vi "XY Graph Set Plot Style.vi"(8 "Error In":errorcluster, 9 "Plot Index (0)":i32, 10 "Single Plot Style":T1, 11 "XY Graph Refnum in":refnum<vi>) -> (0 "Error Out":errorcluster, 3 "XY Graph Refnum out":refnum<vi>)   [LabVIEW 2019, in "XY Graph Add-Ons.lvlib"]
uses:
  XY Graph Add-Ons.lvlib
  Single Plot Style 2.ctl
  Plot Style Settings Step.ctl
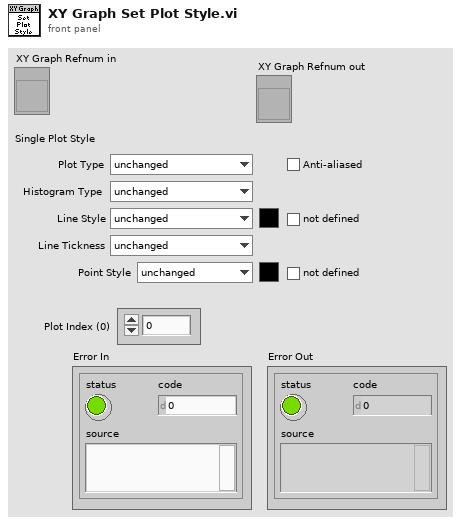
[diagram p1: front panel]
types:
  T1 = typedef "Single Plot Style 2.ctl" = cluster{"Plot Style":enum16{"unchanged", "Line", "Symbol", "Line + Symbol", "Histogram", "Histogram + Symbol"}, "Histogram Type":enum16{"unchanged", "Left Bound", "Center", "Right Bound"}, "Line Tickness":enum16{"unchanged", "Thin", "1 pixel", "2 pixel", "3 pixel", "4 pixel", "5 pixel"}, "Line Style":enum16{"unchanged", "Plain", "Long Dash", "Short Dash", "Long-Short Dash", "Long-Short-Short Dash"}, "Point Style":enum16{"unchanged", "None", "Empty Circle", "Filled Circle", "Thick Circle", "Dotted Circle", "Empty Square", "Filled Square", "Thick Square", "Dotted Square", "Small Filled Square", "Dot", "Cross", "Tiny Cross", "Large X", "Small x", "Diamond", "Small Empty Square"}, "Line Color":u32, "Line Color defined?":bool, "Point Color":u32, "Point Color defined?":bool, "Anti-aliased":bool}
  T2 = typedef "Plot Style Settings Step.ctl" = enum16{"Plot Type", "Line Style", "Line Thickness", "Line Color", "Point Style", "Point Color", "Aliasing"}
  T3 = enum16{"unchanged", "Line", "Symbol", "Line + Symbol", "Histogram", "Histogram + Symbol"}
  T4 = enum16{"unchanged", "Left Bound", "Center", "Right Bound"}
  T5 = enum16{"unchanged", "Plain", "Long Dash", "Short Dash", "Long-Short Dash", "Long-Short-Short Dash"}
  T6 = enum16{"unchanged", "Thin", "1 pixel", "2 pixel", "3 pixel", "4 pixel", "5 pixel"}
  T7 = enum16{"unchanged", "None", "Empty Circle", "Filled Circle", "Thick Circle", "Dotted Circle", "Empty Square", "Filled Square", "Thick Square", "Dotted Square", "Small Filled Square", "Dot", "Cross", "Tiny Cross", "Large X", "Small x", "Diamond", "Small Empty Square"}
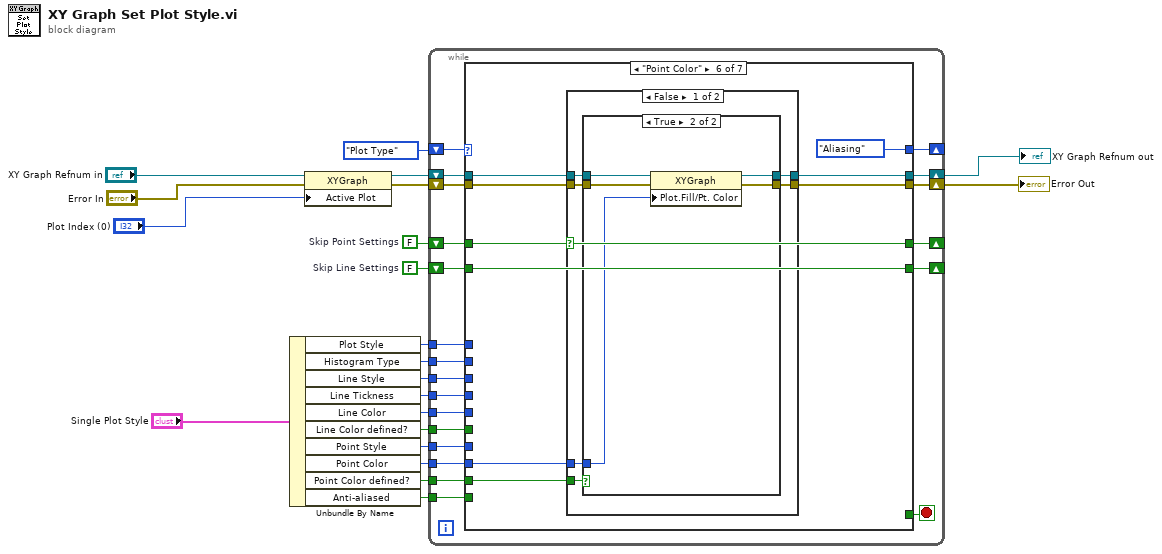
[diagram p0: block diagram]
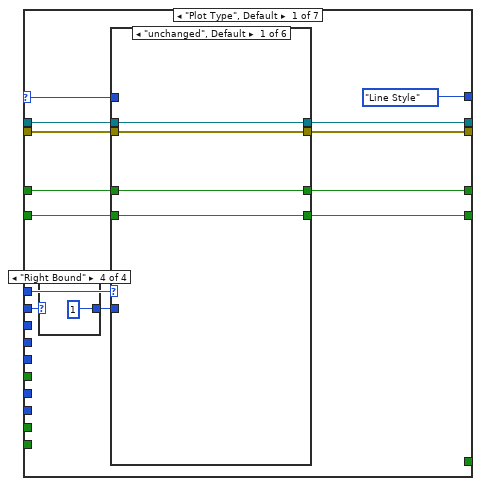
[diagram p2: hidden frame]
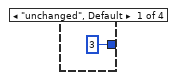
[diagram p3: hidden frame]
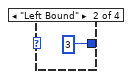
[diagram p4: hidden frame]
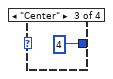
[diagram p5: hidden frame]
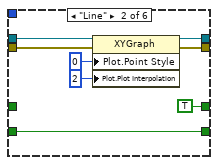
[diagram p6: hidden frame]
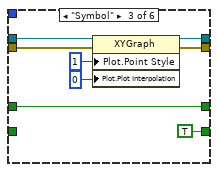
[diagram p7: hidden frame]
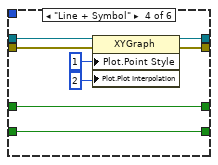
[diagram p8: hidden frame]
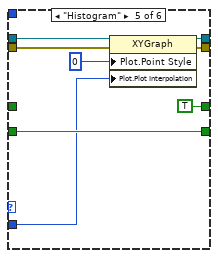
[diagram p9: hidden frame]
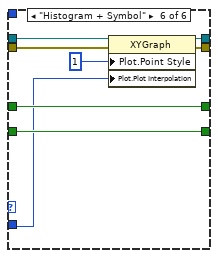
[diagram p10: hidden frame]
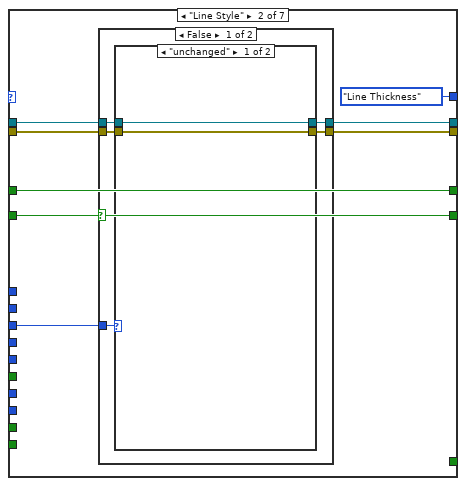
[diagram p11: hidden frame]
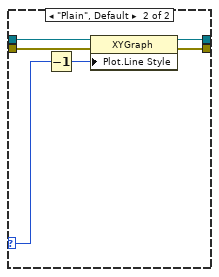
[diagram p12: hidden frame]
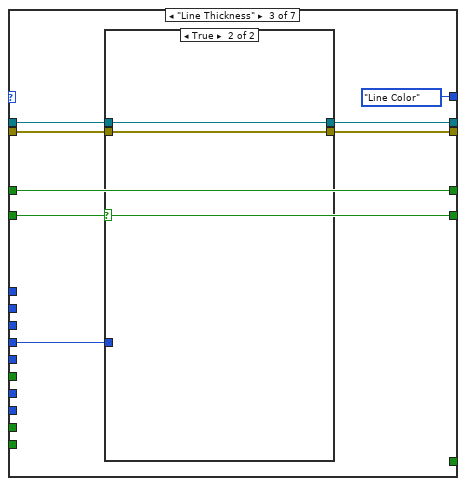
[diagram p14: hidden frame]
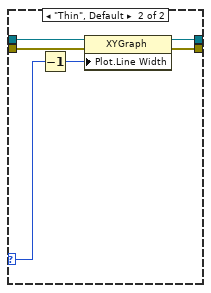
[diagram p16: hidden frame]
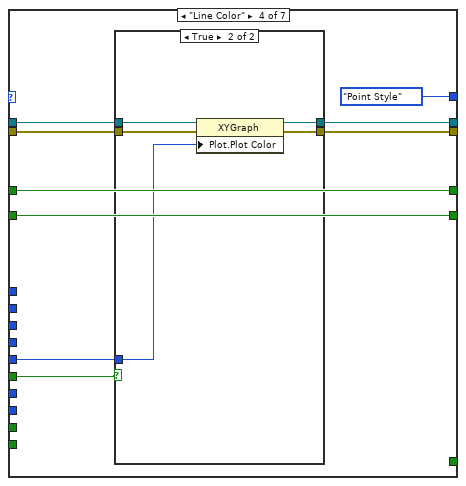
[diagram p17: hidden frame]
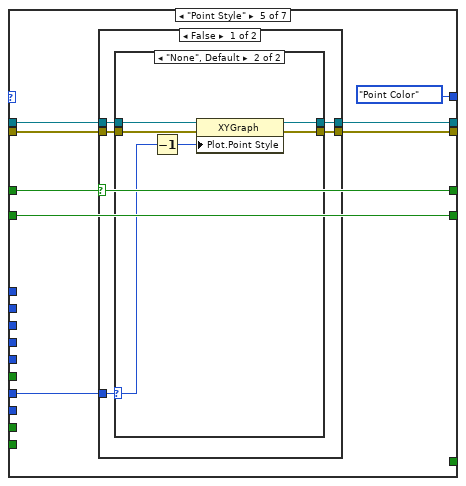
[diagram p19: hidden frame]
diagram:
  w2 = FALSE  # Skip Line Settings
  w3 = FALSE  # Skip Point Settings
  n1 = Unbundle By Name("Single Plot Style") -> ("Plot Style"=w16:T3, "Histogram Type"=w15:T4, "Line Style"=w11:T5, "Line Tickness"=w10:T6, "Line Color"=w9:u32, "Line Color defined?"=w8:bool, "Point Style"=w7:T7, "Point Color"=w5:u32, "Point Color defined?"=w6:bool, "Anti-aliased"=w4:bool)
  n2 = property class="XYGraph"(reference="XY Graph Refnum in", error in="Error In", "Active Plot"="Plot Index (0)") -> (reference out=w14:refnum<vi>, error out=w13:errorcluster)
  n3 = while {
    shift-right: [w37] -> _
    shift-left: Plot_Style_Settings_Step."Plot Type" ("Plot Style Step") -> [w42]
    tunnel: w16 -> [w41]
    tunnel: w15 -> [w40]
    shift-right: [w36] -> w1
    shift-left: w14 -> [w39]
    shift-right: [w35] -> w12
    shift-left: w13 -> [w38]
    tunnel: w11 -> [w34]
    tunnel: w10 -> [w33]
    tunnel: w9 -> [w32]
    tunnel: w8 -> [w31]
    tunnel: w7 -> [w30]
    tunnel: w6 -> [w29]
    tunnel: w5 -> [w28]
    tunnel: w4 -> [w27]
    shift-right: [w24] -> _
    shift-left: w3 -> [w25]
    shift-right: [w22] -> _
    shift-left: w2 -> [w23]
    stop <- w26 stop-if-true
    n4 = case shown="\"Point Color\"" w42 {
      selector: w42 -> [w53 _ _ _ _ _ _]
      tunnel: w41 -> [w55 _ _ _ _ _ _]
      tunnel: w40 -> [w44 _ _ _ _ _ _]
      tunnel: w39 -> [w54 w110 w134 w158 w173 w197 w221]
      tunnel: w38 -> [w52 w108 w132 w156 w171 w195 w219]
      tunnel: [Plot_Style_Settings_Step."Line Style" ("Plot Style Step") Plot_Style_Settings_Step."Line Thickness" ("Plot Style Step") Plot_Style_Settings_Step."Line Color" ("Plot Style Step") Plot_Style_Settings_Step."Point Style" ("Plot Style Step") Plot_Style_Settings_Step."Point Color" ("Plot Style Step") Plot_Style_Settings_Step."Aliasing" ("Plot Style Step") Plot_Style_Settings_Step."Aliasing" ("Plot Style Step")] -> w37
      tunnel: [w50 w109 w133 w157 w172 w196 w220] -> w36
      tunnel: [w49 w107 w131 w155 w170 w194 w218] -> w35
      tunnel: w34 -> [_ w111 _ _ _ _ _]
      tunnel: w33 -> [_ _ w129 _ _ _ _]
      tunnel: w32 -> [_ _ _ w152 _ _ _]
      tunnel: w31 -> [_ _ _ w153 _ _ _]
      tunnel: w30 -> [_ _ _ _ w168 _ _]
      tunnel: w29 -> [_ _ _ _ _ w192 _]
      tunnel: w28 -> [_ _ _ _ _ w191 _]
      tunnel: w27 -> [_ _ _ _ _ _ w216]
      tunnel: [_ _ _ _ _ _ TRUE] -> w26
      tunnel: w25 -> [w48 w105 w128 w151 w167 w190 w214]
      tunnel: [w47 w105 w128 w151 w167 w190 w214] -> w24
      tunnel: w23 -> [w46 w104 w127 w150 w166 w189 w213]
      tunnel: [w45 w104 w127 w150 w166 w189 w213] -> w22
      frame "Plot Type", Default {
        n5 = case shown="\"Right Bound\"" w44 {
          tunnel: [u16 3 ("y") u16 3 ("y") u16 4 ("y") u16 1 ("y")] -> w43
          frame "unchanged", Default {
          }
          frame "Left Bound" {
          }
          frame "Center" {
          }
          frame "Right Bound" {
          }
        }
        n6 = case shown="\"unchanged\", Default" w55 {
          tunnel: w43 -> [_ _ _ _ w88 w96]
          tunnel: w54 -> [w63 w71 w79 w87 w95 w103]
          tunnel: w53 -> [_ _ _ _ _ _]
          tunnel: w52 -> [w62 w69 w77 w85 w93 w101]
          tunnel: [w63 w70 w78 w86 w94 w102] -> w50
          tunnel: [w62 w68 w76 w84 w92 w100] -> w49
          tunnel: w48 -> [w61 _ w73 w82 _ w98]
          tunnel: [w61 TRUE ("Skip Point Settings") w73 w82 TRUE ("Skip Point Settings") w98] -> w47
          tunnel: w46 -> [w60 w65 _ w81 w90 w99]
          tunnel: [w60 w65 TRUE ("Skip Line Settings") w81 w90 w99] -> w45
          frame "unchanged", Default {
          }
          frame "Line" {
            n7 = property class="XYGraph"(reference=w71, error in=w69, "Plot.Point Style"=u8 0, "Plot.Plot Interpolation"=u8 2 ("Plot.Point Style")) -> (reference out=w70:refnum<vi>, error out=w68:errorcluster)
          }
          frame "Symbol" {
            n8 = property class="XYGraph"(reference=w79, error in=w77, "Plot.Point Style"=u8 1, "Plot.Plot Interpolation"=u8 0) -> (reference out=w78:refnum<vi>, error out=w76:errorcluster)
          }
          frame "Line + Symbol" {
            n9 = property class="XYGraph"(reference=w87, error in=w85, "Plot.Point Style"=u8 1, "Plot.Plot Interpolation"=u8 2) -> (reference out=w86:refnum<vi>, error out=w84:errorcluster)
          }
          frame "Histogram" {
            n10 = property class="XYGraph"(reference=w95, error in=w93, "Plot.Point Style"=u8 0, "Plot.Plot Interpolation"=w88) -> (reference out=w94:refnum<vi>, error out=w92:errorcluster)
          }
          frame "Histogram + Symbol" {
            n11 = property class="XYGraph"(reference=w103, error in=w101, "Plot.Point Style"=u8 1, "Plot.Plot Interpolation"=w96) -> (reference out=w102:refnum<vi>, error out=w100:errorcluster)
          }
        }
      }
      frame "Line Style" {
        n12 = case shown="False" w104 {
          tunnel: w111 -> [w116 _]
          tunnel: w110 -> [w115 w126]
          tunnel: [w114 w126] -> w109
          tunnel: w108 -> [w113 w125]
          tunnel: [w112 w125] -> w107
          frame False {
            n13 = case shown="\"unchanged\"" w116 {
              selector: w116 -> [_ w123]
              tunnel: w115 -> [w118 w124]
              tunnel: [w118 w122] -> w114
              tunnel: w113 -> [w117 w120]
              tunnel: [w117 w121] -> w112
              frame "unchanged" {
              }
              frame "Plain", Default {
                n14 = Decrement(x=w123) -> (x-1=w119:T5)
                n15 = property class="XYGraph"(reference=w124, error in=w120, "Plot.Line Style"=w119) -> (reference out=w122:refnum<vi>, error out=w121:errorcluster)
              }
            }
          }
          frame True {
          }
        }
      }
      frame "Line Thickness" {
        n16 = case shown="True" w127 {
          tunnel: w134 -> [w139 w149]
          tunnel: [w138 w149] -> w133
          tunnel: w132 -> [w137 w148]
          tunnel: [w136 w148] -> w131
          tunnel: w129 -> [w135 _]
          frame False {
            n17 = case shown="\"unchanged\"" w135 {
              selector: w135 -> [_ w146]
              tunnel: w139 -> [w141 w147]
              tunnel: [w141 w145] -> w138
              tunnel: w137 -> [w140 w143]
              tunnel: [w140 w144] -> w136
              frame "unchanged" {
              }
              frame "Thin", Default {
                n18 = Decrement(x=w146) -> (x-1=w142:T6)
                n19 = property class="XYGraph"(reference=w147, error in=w143, "Plot.Line Width"=w142) -> (reference out=w145:refnum<vi>, error out=w144:errorcluster)
              }
            }
          }
          frame True {
          }
        }
      }
      frame "Line Color" {
        n20 = case shown="True" w153 {
          tunnel: w158 -> [w160 w165]
          tunnel: [w160 w164] -> w157
          tunnel: w156 -> [w159 w162]
          tunnel: [w159 w163] -> w155
          tunnel: w152 -> [_ w161]
          frame False {
          }
          frame True {
            n21 = property class="XYGraph"(reference=w165, error in=w162, "Plot.Plot Color"=w161) -> (reference out=w164:refnum<vi>, error out=w163:errorcluster)
          }
        }
      }
      frame "Point Style" {
        n22 = case shown="False" w167 {
          tunnel: w173 -> [w178 w188]
          tunnel: [w177 w188] -> w172
          tunnel: w171 -> [w176 w187]
          tunnel: [w175 w187] -> w170
          tunnel: w168 -> [w174 _]
          frame False {
            n23 = case shown="\"None\", Default" w174 {
              selector: w174 -> [_ w185]
              tunnel: w178 -> [w180 w186]
              tunnel: [w180 w184] -> w177
              tunnel: w176 -> [w179 w182]
              tunnel: [w179 w183] -> w175
              frame "unchanged" {
              }
              frame "None", Default {
                n24 = Decrement(x=w185) -> (x-1=w181:T7)
                n25 = property class="XYGraph"(reference=w186, error in=w182, "Plot.Point Style"=w181) -> (reference out=w184:refnum<vi>, error out=w183:errorcluster)
              }
            }
          }
          frame True {
          }
        }
      }
      frame "Point Color" {
        n26 = case shown="False" w190 {
          tunnel: w197 -> [w203 w212]
          tunnel: [w202 w212] -> w196
          tunnel: w195 -> [w201 w211]
          tunnel: [w200 w211] -> w194
          tunnel: w192 -> [w199 _]
          tunnel: w191 -> [w198 _]
          frame False {
            n27 = case shown="True" w199 {
              tunnel: w203 -> [w205 w210]
              tunnel: [w205 w209] -> w202
              tunnel: w201 -> [w204 w207]
              tunnel: [w204 w208] -> w200
              tunnel: w198 -> [_ w206]
              frame False {
              }
              frame True {
                n28 = property class="XYGraph"(reference=w210, error in=w207, "Plot.Fill/Pt. Color"=w206) -> (reference out=w209:refnum<vi>, error out=w208:errorcluster)
              }
            }
          }
          frame True {
          }
        }
      }
      frame "Aliasing" {
        n29 = property class="XYGraph"(reference=w221, error in=w219, "Plot.Anti-aliased"=w216) -> (reference out=w220:refnum<vi>, error out=w218:errorcluster)
      }
    }
  }
  "Error Out" <- w12
  "XY Graph Refnum out" <- w1
